vi "Open Sysdef Refs for IP Set.vi"(8 "error in (no error)":errorcluster, 11 "UUT Path":path) -> (0 "error out":errorcluster, 1 "Targets":refnum<k24>[](array[refnum]), 2 "SysDef":refnum<k24>, 3 "UUT Path":path)   [LabVIEW 2011]
uses:
  NationalInstruments.VeriStand.SystemDefinitionAPI
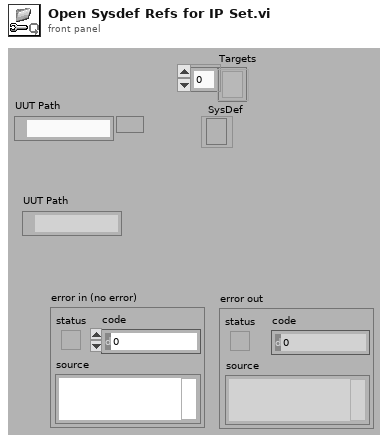
[diagram p1: front panel]
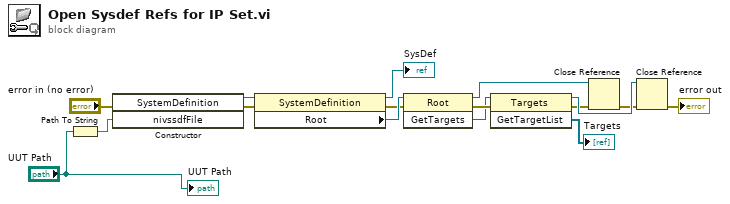
[diagram p0: block diagram]
diagram:
  n1 = Path To String(path="UUT Path") -> (string=w13:string)
  n2 = constructor class="SystemDefinition"(error in="error in (no error)", "nivssdfFile"=w13) -> (reference out=w16:refnum<k24>, error out=w15:errorcluster)  [unwired: 2 in, 2 out]
  n3 = property class="SystemDefinition"(reference=w16, error in=w15) -> (reference out=→"SysDef":refnum<k24>, error out=w9:errorcluster, "Root"=w10:refnum<k24>)
  n4 = invoke class="Root" method="GetTargets"(reference=w10, error in=w9) -> (reference out=w7:refnum<k24>, error out=w8:errorcluster, "GetTargets"=w6:refnum<k24>)  [unwired: 1 in]
  n5 = invoke class="Targets" method="GetTargetList"(reference=w6, error in=w8) -> (reference out=w12:refnum<k24>, error out=w4:errorcluster, "GetTargetList"=→"Targets":refnum<k24>[])  [unwired: 1 in]
  n6 = Close Reference(reference=w7, error in (no error)=w4) -> (error out=w11:errorcluster)
  n7 = Close Reference(reference=w12, error in (no error)=w11) -> (error out=→"error out":errorcluster)
  "UUT Path" <- "UUT Path"
